vi "obj_DataLog Tag Meta Tags.vi"(0 "method":T3, 7 "point to write":T2 {"value" format="%.3e"; "time" format="%<%H:%M:%S%2u\n%Y/%m/%d>T"}, 9 "tag index in":i32=-1, 11 "error in (no error)":errorcluster) -> (4 "limit events":T1[](array[typedef]), 6 "exceeded mask":u32 format="%.0b", 8 "meta tag indices (-1 if none)":i32[](array[numeric]), 10 "tag index dup":i32, 15 "error out":errorcluster)   [LabVIEW 2012]
doc: "This object serves to apply meta tags to points being written to tags with direct valuation. Since only existing meta tags require application, the meta tags are collected on initialization so that their existence can be quickly determined. The max/min bounds are applied when exceeded. Subsequently, exceeded limits cause corresponding flags to be set, but the events are triggered conditionally based on the tag configuration settings intended to supress spurious events. Also, events are not handled by this non-reentrant object so as to prevent contention (event handling can be expensive). To ensure limit event handling, this object's {apply and write} method may not be called directly. Instead the \"Check and Write Point\" reentrant VI should be used since, in addition to calling {apply and write}, it implements event handling without contention.\n\nSince the {apply and write} method is called very frequently, some effort was put into minimizing its average overhead by putting most checking code on the same diagram (wich prevents subVI calling overhead) as well as by deferring object calls as long as possible by first checking for necessity. Hence the rather large diagram."
uses:
  typedefs/t_DataLog Tag Meta Tags Methods.ctl
  typedefs/et_DataLog Meta Tag Specifier.ctl
  typedefs/clusters/t_DataLog Point.ctl
  typedefs/t_DataLog Tag Hash Methods.ctl
  typedefs/t_DataLog Tag Info List Methods.ctl
  typedefs/t_DataLog Tag Buffers Methods.ctl
  subvis/private/glb_DataLog Runtime Parameterisation.vi
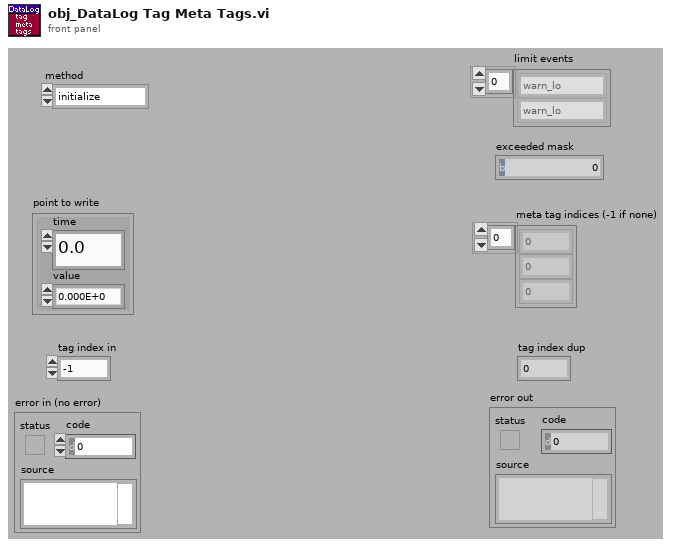
[diagram p1: front panel]
types:
  T1 = typedef "et_DataLog Meta Tag Specifier.ctl" = enum32{"warn_lo", "warn_hi", "A_lo", "A_hi", "B_lo", "B_hi", "C_lo", "C_hi", "D_lo", "D_hi", "E_lo", "E_hi", "F_lo", "F_hi", "G_lo", "G_hi", "H_lo", "H_hi", "I_lo", "I_hi", "J_lo", "J_hi", "K_lo", "K_hi", "L_lo", "L_hi", "M_lo", "M_hi", "N_lo", "N_hi", "min", "max", "not a meta"}
  T2 = typedef "t_DataLog Point.ctl" = cluster{"time":dbl, "value":dbl}
  T3 = typedef "t_DataLog Tag Meta Tags Methods.ctl" = enum16{"initialize", "apply and write", "get exceeded", "get metas", "cleanup"}
  T4 = typedef "t_DataLog Tag Hash Methods.ctl" = enum16{"initialize", "add tag", "index tag", "lookup", "#tags", "cleanup", "write recovery", "read recovery", "delete recovery"}
  T5 = typedef "t_DataLog Tag Info List Methods.ctl" = enum16{"initialize", "create", "create empty", "rename", "delete", "test tag", "get", "get by name", "get default", "get list", "get path", "get subsets", "set subsets", "set config", "set capacity", "#tags", "go live", "set unlocked", "set mirrored"}
  T6 = typedef "t_DataLog Tag Buffers Methods.ctl" = enum16{"initialize", "inert", "write", "read", "read oldest", "read last", "cleanup"}
  T7 = typedef "t_DataLog Tag Config.ctl" = cluster{"name":string, "unit":string, "temporal":T8, "value":T9, "index":i32, "capacity":i32, "is meta?":bool, "mincapacity":i32, "deadband":dbl, "limit delay":dbl, "format":T10, "precision":u8, "undefine":bool, "update":bool, "update period":u16, "expression":string, "description":string, "logging algorithm":T11, "logging parameters":dbl[]}
  T8 = typedef "t_DataLog Temporal Types.ctl" = enum16{"set&hold", "sample", "event"}
  T9 = typedef "t_DataLog Value Types.ctl" = enum16{"number", "string"}
  T10 = typedef "t_DataLog Numerical Format.ctl" = enum8{"fractional", "exponential", "engineering"}
  T11 = typedef "t_DataLog Logging Algorithms.ctl" = enum16{"nothing", "changes", "everything", "every Nth", "time threshold", "value threshold + prior", "t or v threshold", "t or v threshold + prior"}
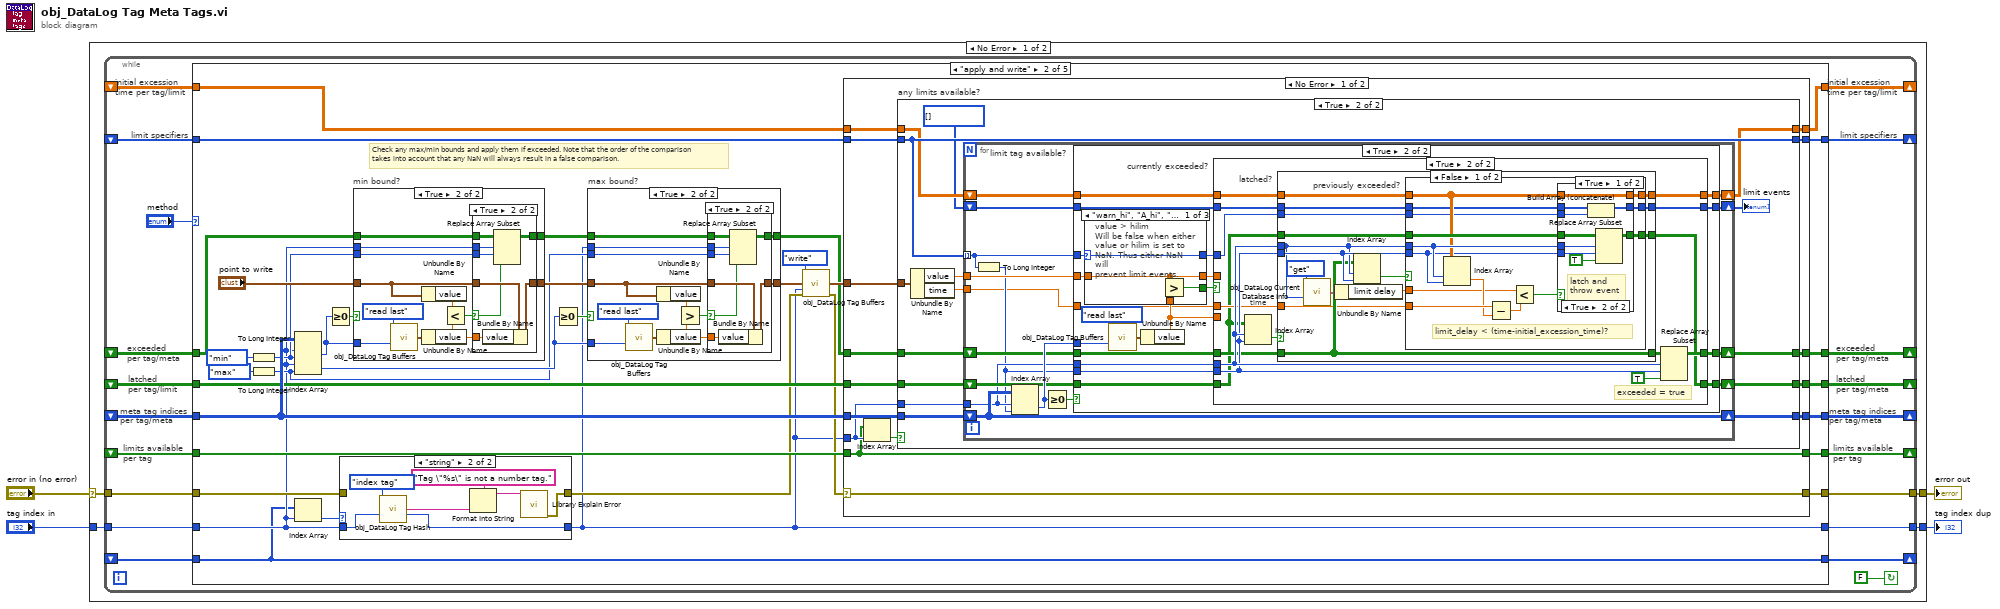
[diagram p0: block diagram]
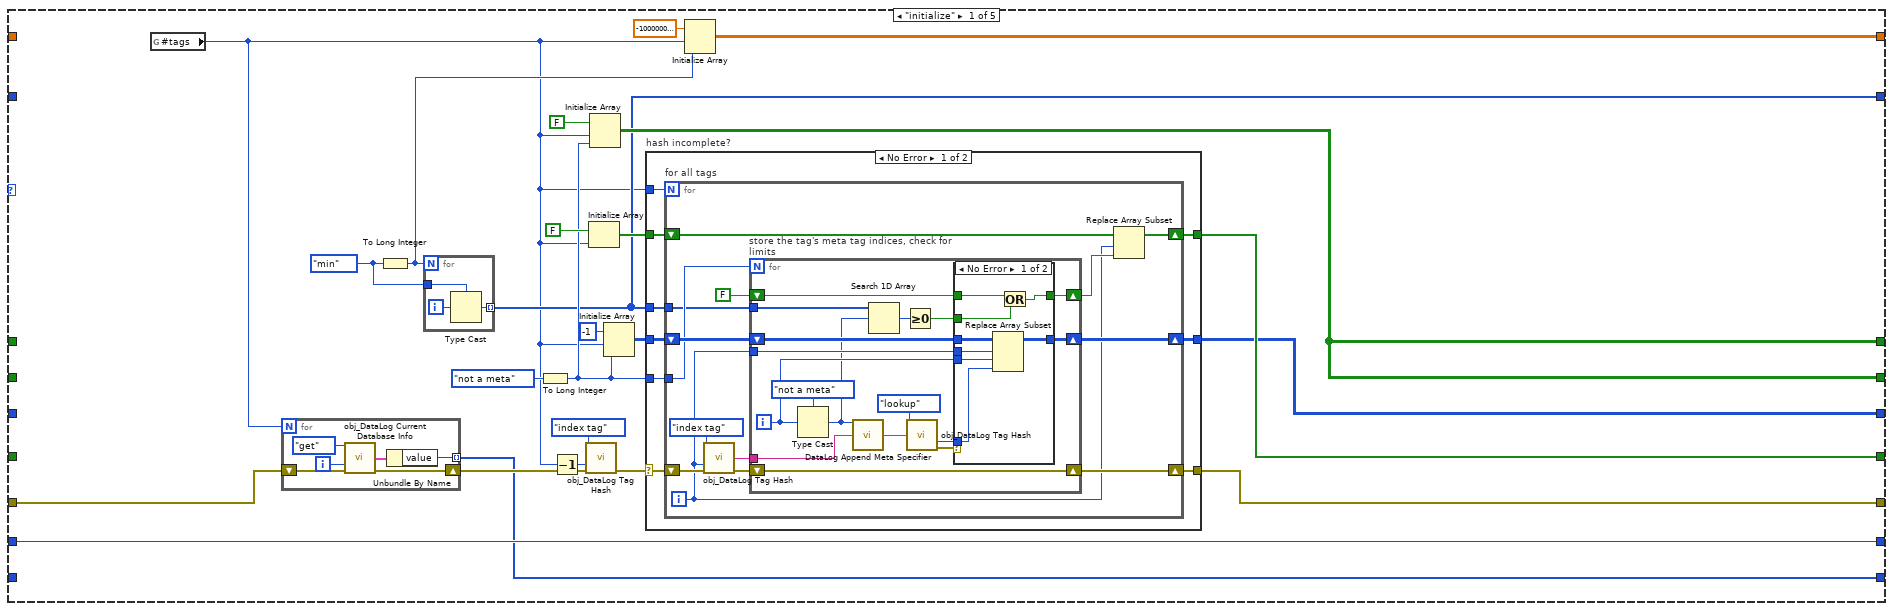
[diagram p2: hidden frame]
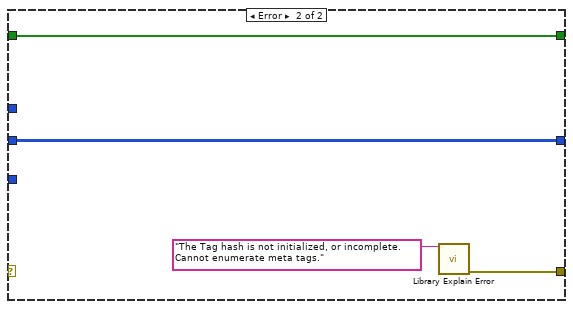
[diagram p4: hidden frame]
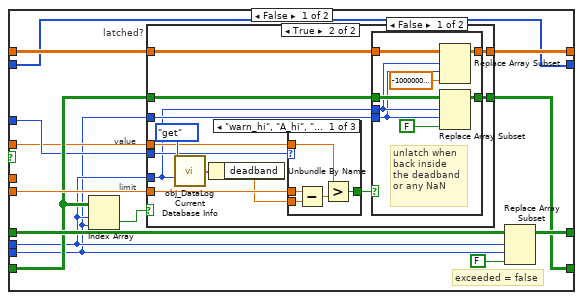
[diagram p8: hidden frame]
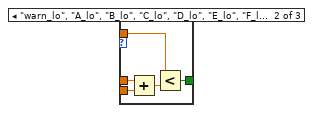
[diagram p11: hidden frame]
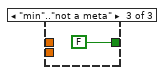
[diagram p12: hidden frame]
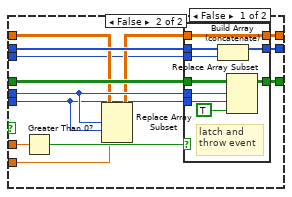
[diagram p14: hidden frame]
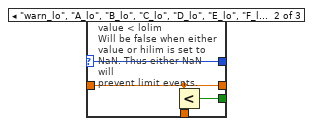
[diagram p17: hidden frame]
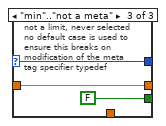
[diagram p18: hidden frame]
diagram:
  n1 = case shown="No Error" "error in (no error)" {
    selector: "error in (no error)" -> [w8 w581]
    tunnel: [w7 w581] -> w3
    tunnel: [w6 w580] -> w2
    tunnel: "tag index in" -> [w5 w580]
    frame No Error {
      n2 = while {
        shift-right: [w26] -> _
        shift-left: _ -> [w25]
        tunnel: w8 -> [w24]
        tunnel: [w23] -> w7
        shift-right: [w21] -> _
        shift-left: _ -> [w22]
        shift-right: [w19] -> _
        shift-left: _ -> [w20]
        shift-right: [w17] -> _
        shift-left: _ -> [w18]
        shift-right: [w15] -> _
        shift-left: _ -> [w16]
        shift-right: [w14] -> _
        shift-left: _ -> [w13]
        shift-right: [w12] -> _
        shift-left: _ -> [w11]
        tunnel: [w10] -> w6
        tunnel: w5 -> [w9]
        stop <- FALSE continue-if-true
        # "initial excession\ntime per tag/limit"
        # "limit specifiers"
        # "limits available\nper tag"
        # "exceeded\nper tag/meta"
        # "latched\nper tag/meta"
        # "meta tag indices\nper tag/meta"
        # "exceeded\nper tag/meta"
        # "latched\nper tag/meta"
        # "exceeded\nper tag/meta"
        # "initial excession\ntime per tag/limit"
        # "exceeded\nper tag/meta"
        # "limit specifiers"
        # "latched\nper tag/limit"
        # "limits available\nper tag"
        # "meta tag indices\nper tag/meta"
        n3 = case shown="\"apply and write\"" "method" {
          tunnel: w25 -> [_ w149 w456 w536 w571]
          tunnel: [w48 w148 w449 w529 w568] -> w26
          tunnel: w24 -> [w31 w121 w458 w538 w579]
          tunnel: [w51 w132 w460 w540 w579] -> w23
          tunnel: w22 -> [_ w150 w447 w527 w573]
          tunnel: [w50 w131 w457 w537 w572] -> w21
          tunnel: w20 -> [_ w146 w452 w532 w570]
          tunnel: [w39 w147 w455 w535 w569] -> w19
          tunnel: w9 -> [w41 w118 w454 w534 w578]
          tunnel: [w41 w119 w453 w533 w578] -> w10
          tunnel: w18 -> [_ w145 w446 w526 w577]
          tunnel: [w35 w144 w445 w526 w575] -> w17
          tunnel: w16 -> [_ w126 w451 w531 w564]
          tunnel: [w39 w130 w450 w530 w563] -> w15
          tunnel: [w38 w142 w448 w528 w561] -> w14
          tunnel: w13 -> [_ w143 w448 w528 w562]
          tunnel: [w29 w117 w444 w525 w557] -> w12
          tunnel: w11 -> [_ w117 w444 w525 w558]
          frame "initialize" {
            w34 = et_DataLog_Meta_Tag_Specifier."min" ("meta specifier")
            n4 = global read "glb_DataLog Runtime Parameterisation.vi" "#tags"() -> (w32:i32)
            n5 = for {
              N: w32 -> [_]
              shift-right: [w54] -> w30
              shift-left: w31 -> [w55]
              tunnel: [w53] -> w29 mode=indexing
              i -> [w56]
              n6 = call "obj_DataLog Current Database Info.vi"("method"=t_DataLog_Tag_Info_List_Methods."get", "tag index/change#"=w56, "error in (no error)"=w55) -> ("tag config out"=w57:T7, "error out"=w54:errorcluster)  [unwired: 6 in, 5 out]
              n7 = Unbundle By Name(w57) -> ("value"=w53:T9)
            }
            n8 = To Long Integer(number=w34) -> (32bit integer=w33:i32)
            n9 = for {
              N: w33 -> [_]
              tunnel: w34 -> [w61]
              tunnel: [w59] -> w35 mode=indexing
              i -> [w60]
              n10 = Type Cast(type=w61, x=w60) -> (*(type *) &x=w59:T1)
            }
            n11 = To Long Integer(number=et_DataLog_Meta_Tag_Specifier."not a meta" ("limit specifier")) -> (32bit integer=w36:i32)
            n12 = Decrement(x=w32) -> (x-1=w47:i32)
            n13 = call "obj_DataLog Tag Hash.vi"("method"=t_DataLog_Tag_Hash_Methods."index tag", "tag index in"=w47, "error in (no error)"=w30) -> ("error out"=w45:errorcluster)  [unwired: 9 in, 3 out]
            n14 = Initialize Array(FALSE, w32) -> (w49:bool[])
            n15 = Initialize Array(FALSE, w32, w36) -> (w39:bool[][])
            n16 = Initialize Array(-1 ("warning lolim"), w32, w36) -> (w43:i32[][])
            n17 = case "hash incomplete?" shown="No Error" w45 {
              selector: w45 -> [w64 _]
              tunnel: w32 -> [w70 _]
              tunnel: [w65 w112] -> w51
              tunnel: [w69 w115] -> w50
              tunnel: w49 -> [w68 w115]
              tunnel: [w67 w114] -> w48
              tunnel: w43 -> [w66 w114]
              tunnel: w36 -> [w63 _]
              tunnel: w35 -> [w62 _]
              frame No Error {
                n18 = for "for all tags" {
                  N: w70 -> [_]
                  shift-right: [w78] -> w69
                  shift-left: w68 -> [w77]
                  shift-right: [w75] -> w67
                  shift-left: w66 -> [w76]
                  shift-right: [w81] -> w65
                  shift-left: w64 -> [w83]
                  tunnel: w63 -> [w74]
                  tunnel: w62 -> [w71]
                  i -> [w72]
                  n19 = call "obj_DataLog Tag Hash.vi"("method"=t_DataLog_Tag_Hash_Methods."index tag", "tag index in"=w72, "error in (no error)"=w83) -> ("tag out"=w80:string, "error out"=w82:errorcluster)  [unwired: 9 in, 2 out]
                  n20 = for "store the tag's meta tag indices, check for limits" {
                    N: w74 -> [_]
                    shift-right: [w86] -> w81
                    shift-left: w82 -> [w86]
                    tunnel: w80 -> [w97]
                    shift-right: [w100] -> w75
                    shift-left: w76 -> [w101]
                    shift-right: [w98] -> w73
                    shift-left: FALSE -> [w99]
                    tunnel: w72 -> [w91]
                    tunnel: w71 -> [w89]
                    i -> [w90]
                    n21 = Type Cast(type=et_DataLog_Meta_Tag_Specifier."not a meta" ("limit specifier"), x=w90) -> (*(type *) &x=w85:T1)
                    n22 = call "DataLog Append Meta Specifier.vi"("meta specifier"=w85, "tag in"=w97) -> ("tag out"=w95:string)  [unwired: 13 in]
                    n23 = Search 1D Array(1D array=w89, element=w85) -> (index of element=w88:i32)  [unwired: 1 in]
                    n24 = Greater Or Equal To 0?(x=w88) -> (x >= 0?=w87:bool)
                    n25 = call "obj_DataLog Tag Hash.vi"("method"=t_DataLog_Tag_Hash_Methods."lookup", "tag in"=w95) -> ("tag index out"=w93:i32, "error out"=w92:errorcluster)  [unwired: 10 in, 2 out]
                    n26 = case shown="No Error" w92 {
                      tunnel: w101 -> [w108 w110]
                      tunnel: [w107 w110] -> w100
                      tunnel: w99 -> [w103 w111]
                      tunnel: [w109 w111] -> w98
                      tunnel: w93 -> [w106 _]
                      tunnel: w91 -> [w105 _]
                      tunnel: w90 -> [w104 _]
                      tunnel: w87 -> [w102 _]
                      frame No Error {
                        n27 = Replace Array Subset(array=w108, new element=w106, index (row)=w105, index (col)=w104) -> (w107:i32[][])
                        n28 = Or(x=w103, y=w102) -> (x .or. y?=w109:bool)
                      }
                      frame Error {
                      }
                    }
                  }
                  n29 = Replace Array Subset(array=w77, new element=w73, index=w72) -> (w78:bool[])
                }
              }
              frame Error {
                n30 = call "Library Explain Error.vi"("explanation prefix (none)"="The Tag hash is not initialized, or incomplete. Cannot enumerate meta tags." ("explanation")) -> ("explained error"=w112:errorcluster)  [unwired: 14 in]
              }
            }
            n31 = Initialize Array(-1000000000000.0, w32, w33) -> (w38:dbl[][])
          }
          frame "apply and write" {
            # "Check any max/min bounds and apply them if exceeded. Note that the order of the comparison takes into account that any NaN will always result in a false comparison."
            n32 = To Long Integer(number=et_DataLog_Meta_Tag_Specifier."min" ("meta specifier")) -> (32bit integer=w122:i32)
            n33 = To Long Integer(number=et_DataLog_Meta_Tag_Specifier."max" ("meta specifier")) -> (32bit integer=w125:i32)
            n34 = Index Array(array=w149, index (row) #1=w118, index (col) #1=w122, index (row) #2=w118, index (col) #2=w125) -> (element #1=w137:i32, element #2=w129:i32)
            n35 = Index Array(array=w117, index=w118) -> (element=w116:T9)
            n36 = Greater Or Equal To 0?(x=w137) -> (x >= 0?=w136:bool)
            n37 = case shown="\"string\"" w116 {
              tunnel: w121 -> [w152 _]
              tunnel: [w152 w155] -> w120
              tunnel: w118 -> [w151 w154]
              tunnel: [w151 w153] -> w119
              frame "number" {
              }
              frame "string" {
                n38 = call "obj_DataLog Tag Hash.vi"("method"=t_DataLog_Tag_Hash_Methods."index tag", "tag index in"=w154) -> ("tag out"=w156:string, "tag index out"=w153:i32)  [unwired: 10 in, 2 out]
                n39 = Format Into String(format string="Tag \"%s\" is not a number tag.", w156) -> (resulting string=w157:string)  [unwired: 2 in, 1 out]
                n40 = call "Library Explain Error.vi"("explanation prefix (none)"=w157) -> ("explained error"=w155:errorcluster)  [unwired: 14 in]
              }
            }
            n41 = case "min bound?" shown="True" w136 {
              tunnel: w137 -> [_ w427]
              tunnel: "point to write" -> [w417 w423]
              tunnel: [w417 w422] -> w128
              tunnel: w126 -> [w416 w421]
              tunnel: w118 -> [_ w420]
              tunnel: [w416 w419] -> w124
              tunnel: w122 -> [_ w418]
              frame False {
              }
              frame True {
                n42 = call "obj_DataLog Tag Buffers.vi"("method"=t_DataLog_Tag_Buffers_Methods."read last", "tag index"=w427) -> ("point out"=w429:T2)  [unwired: 9 in, 4 out]
                n43 = Unbundle By Name(w423) -> ("value"=w426:dbl)
                n44 = Unbundle By Name(w429) -> ("value"=w425:dbl)
                n45 = Less?(x=w426, y=w425) -> (x < y?=w424:bool)
                n46 = case shown="True" w424 {
                  selector: w424 -> [w433 w436]
                  tunnel: w423 -> [w435 w443]
                  tunnel: w425 -> [_ w441]
                  tunnel: [w435 w442] -> w422
                  tunnel: w421 -> [w434 w440]
                  tunnel: w420 -> [w431 w439]
                  tunnel: [w430 w438] -> w419
                  tunnel: w418 -> [w432 w437]
                  frame False {
                    n47 = Replace Array Subset(array=w434, new element=w433, index (row)=w431, index (col)=w432) -> (w430:bool[][])
                  }
                  frame True {
                    n48 = Bundle By Name(cluster=w443, "value"=w441) -> (w442:T2)
                    n49 = Replace Array Subset(array=w440, new element=w436, index (row)=w439, index (col)=w437) -> (w438:bool[][])
                  }
                }
              }
            }
            n50 = Greater Or Equal To 0?(x=w129) -> (x >= 0?=w135:bool)
            n51 = case "max bound?" shown="True" w135 {
              tunnel: w129 -> [_ w399]
              tunnel: w128 -> [w389 w395]
              tunnel: [w389 w394] -> w134
              tunnel: w119 -> [_ w393]
              tunnel: w124 -> [w388 w392]
              tunnel: w125 -> [_ w391]
              tunnel: [w388 w390] -> w123
              frame False {
              }
              frame True {
                n52 = call "obj_DataLog Tag Buffers.vi"("method"=t_DataLog_Tag_Buffers_Methods."read last", "tag index"=w399) -> ("point out"=w401:T2)  [unwired: 9 in, 4 out]
                n53 = Unbundle By Name(w395) -> ("value"=w398:dbl)
                n54 = Unbundle By Name(w401) -> ("value"=w397:dbl)
                n55 = Greater?(x=w398, y=w397) -> (0:w396:bool)
                n56 = case shown="True" w396 {
                  selector: w396 -> [w403 w411]
                  tunnel: w395 -> [w407 w415]
                  tunnel: w397 -> [_ w413]
                  tunnel: [w407 w414] -> w394
                  tunnel: w393 -> [w405 w412]
                  tunnel: w392 -> [w406 w410]
                  tunnel: w391 -> [w404 w409]
                  tunnel: [w402 w408] -> w390
                  frame False {
                    n57 = Replace Array Subset(array=w406, new element=w403, index (row)=w405, index (col)=w404) -> (w402:bool[][])
                  }
                  frame True {
                    n58 = Bundle By Name(cluster=w415, "value"=w413) -> (w414:T2)
                    n59 = Replace Array Subset(array=w410, new element=w411, index (row)=w412, index (col)=w409) -> (w408:bool[][])
                  }
                }
              }
            }
            n60 = call "obj_DataLog Tag Buffers.vi"("method"=t_DataLog_Tag_Buffers_Methods."write", "point in"=w134, "tag index"=w119, "error in (no error)"=w120) -> ("point out"=w140:T2, "error out"=w133:errorcluster)  [unwired: 7 in, 3 out]
            n61 = case shown="No Error" w133 {
              selector: w133 -> [w162 w387]
              tunnel: w150 -> [w161 w386]
              tunnel: w149 -> [w174 w385]
              tunnel: [w173 w385] -> w148
              tunnel: [w172 w384] -> w147
              tunnel: w146 -> [w171 w384]
              tunnel: w123 -> [w170 w381]
              tunnel: w145 -> [w169 w382]
              tunnel: [w168 w382] -> w144
              tunnel: w143 -> [w167 w383]
              tunnel: [w166 w383] -> w142
              tunnel: w119 -> [w165 _]
              tunnel: w140 -> [w163 _]
              tunnel: [w162 w387] -> w132
              tunnel: [w161 w386] -> w131
              tunnel: [w160 w381] -> w130
              frame No Error {
                n62 = Index Array(array=w161, index=w165) -> (element=w164:bool)
                n63 = case "any limits available?" shown="True" w164 {
                  tunnel: w174 -> [w178 w193]
                  tunnel: w171 -> [w179 w188]
                  tunnel: w163 -> [_ w194]
                  tunnel: [w179 w186] -> w172
                  tunnel: [w178 w192] -> w173
                  tunnel: w165 -> [_ w189]
                  tunnel: w169 -> [w177 w190]
                  tunnel: [w177 w190] -> w168
                  tunnel: w170 -> [w175 w187]
                  tunnel: w167 -> [w176 w183]
                  tunnel: [w176 w182] -> w166
                  tunnel: [w175 w185] -> w160
                  frame False {
                  }
                  frame True {
                    w181 = T1[] [] items=["warn_lo", "warn_hi", "A_lo", "A_hi", "B_lo", "B_hi", "C_lo", "C_hi", "D_lo", "D_hi", "E_lo", "E_hi", "F_lo", "F_hi", "G_lo", "G_hi", "H_lo", "H_hi", "I_lo", "I_hi", "J_lo", "J_hi", "K_lo", "K_hi", "L_lo", "L_hi", "M_lo", "M_hi", "N_lo", "N_hi", "min", "max", "not a meta"] ("limit events")
                    n64 = Unbundle By Name(w194) -> ("value"=w184:dbl, "time"=w191:dbl)
                    n65 = for {
                      shift-right: [w210] -> w192
                      shift-left: w193 -> [w210]
                      tunnel: w191 -> [w197]
                      tunnel: w190 -> [w207] mode=indexing
                      tunnel: w189 -> [w199]
                      shift-right: [w200] -> w186
                      shift-left: w188 -> [w206]
                      shift-right: [w201] -> w185
                      shift-left: w187 -> [w204]
                      tunnel: w184 -> [w205]
                      shift-right: [w202] -> w182
                      shift-left: w183 -> [w203]
                      shift-right: [w195] -> w180
                      shift-left: w181 -> [w196]
                      n66 = To Long Integer(number=w207) -> (32bit integer=w198:i32)
                      n67 = Index Array(array=w210, index (row)=w199, index (col)=w198) -> (element=w209:i32)
                      n68 = Greater Or Equal To 0?(x=w209) -> (x >= 0?=w208:bool)
                      n69 = case "limit tag available?" shown="True" w208 {
                        tunnel: w207 -> [_ w231]
                        tunnel: w209 -> [_ w234]
                        tunnel: w206 -> [w212 w227]
                        tunnel: w205 -> [_ w230]
                        tunnel: w204 -> [w213 w228]
                        tunnel: w203 -> [w214 w226]
                        tunnel: [w214 w225] -> w202
                        tunnel: [w213 w224] -> w201
                        tunnel: [w212 w221] -> w200
                        tunnel: w199 -> [_ w223]
                        tunnel: w198 -> [_ w222]
                        tunnel: w197 -> [_ w217]
                        tunnel: w196 -> [w211 w216]
                        tunnel: [w211 w215] -> w195
                        frame False {
                        }
                        frame True {
                          n70 = call "obj_DataLog Tag Buffers.vi"("method"=t_DataLog_Tag_Buffers_Methods."read last", "tag index"=w234) -> ("point out"=w232:T2)  [unwired: 9 in, 4 out]
                          n71 = Unbundle By Name(w232) -> ("value"=w219:dbl)
                          n72 = case shown="\"warn_hi\", \"A_hi\", \"B_hi\", \"C_hi\", \"D_hi\", \"E_hi\", \"F_hi\", \"G_hi\", \"H_hi\", \"I_hi\", \"J_hi\", \"K_hi\", \"L_hi\", \"M_hi\", \"N_hi\"" w231 {
                            selector: w231 -> [w370 w374 w378]
                            tunnel: w230 -> [w371 w375 w379]
                            tunnel: w219 -> [w373 w377 _]
                            tunnel: [w372 w376 FALSE] -> w229
                            tunnel: [w371 w375 w379] -> w220
                            tunnel: [w370 w374 w378] -> w218
                            frame "warn_hi", "A_hi", "B_hi", "C_hi", "D_hi", "E_hi", "F_hi", "G_hi", "H_hi", "I_hi", "J_hi", "K_hi", "L_hi", "M_hi", "N_hi" {
                              # "value > hilim\nWill be false when either value or hilim is set to NaN. Thus either NaN will\nprevent limit events."
                              n73 = Greater?(x=w371, y=w373) -> (0:w372:bool)
                            }
                            frame "warn_lo", "A_lo", "B_lo", "C_lo", "D_lo", "E_lo", "F_lo", "G_lo", "H_lo", "I_lo", "J_lo", "K_lo", "L_lo", "M_lo", "N_lo" {
                              # "value < lolim\nWill be false when either value or hilim is set to NaN. Thus either NaN will\nprevent limit events."
                              n74 = Less?(x=w375, y=w377) -> (x < y?=w376:bool)
                            }
                            frame "min".."not a meta" {
                              # "not a limit, never selected\nno default case is used to\nensure this breaks on modification of the meta\ntag specifier typedef"
                            }
                          }
                          n75 = case "currently exceeded?" shown="True" w229 {
                            tunnel: w228 -> [w248 w287]
                            tunnel: w227 -> [w243 w285]
                            tunnel: w226 -> [w236 w293]
                            tunnel: [w237 w292] -> w225
                            tunnel: [w247 w299] -> w224
                            tunnel: w223 -> [w241 w295]
                            tunnel: w222 -> [w238 w294]
                            tunnel: [w242 w296] -> w221
                            tunnel: w220 -> [w239 _]
                            tunnel: w219 -> [w244 _]
                            tunnel: w218 -> [w240 w289]
                            tunnel: w217 -> [_ w291]
                            tunnel: w216 -> [w235 w290]
                            tunnel: [w235 w288] -> w215
                            frame False {
                              # "exceeded = false"
                              # "limit"
                              # "value"
                              n76 = Index Array(array=w243, index (row)=w241, index (col)=w238) -> (element=w245:bool)
                              n77 = case "latched?" shown="True" w245 {
                                tunnel: w244 -> [_ w259]
                                tunnel: w243 -> [w250 w256]
                                tunnel: [w250 w255] -> w242
                                tunnel: w241 -> [_ w253]
                                tunnel: w240 -> [_ w261]
                                tunnel: w239 -> [_ w260]
                                tunnel: w238 -> [_ w254]
                                tunnel: [w249 w252] -> w237
                                tunnel: w236 -> [w249 w251]
                                frame False {
                                }
                                frame True {
                                n78 = call "obj_DataLog Current Database Info.vi"("method"=t_DataLog_Tag_Info_List_Methods."get", "tag index/change#"=w253) -> ("tag config out"=w262:T7)  [unwired: 7 in, 6 out]
                                n79 = Unbundle By Name(w262) -> ("deadband"=w258:dbl)
                                n80 = case shown="\"warn_hi\", \"A_hi\", \"B_hi\", \"C_hi\", \"D_hi\", \"E_hi\", \"F_hi\", \"G_hi\", \"H_hi\", \"I_hi\", \"J_hi\", \"K_hi\", \"L_hi\", \"M_hi\", \"N_hi\"" w261 {
                                tunnel: [w278 w283 FALSE] -> w257
                                tunnel: w260 -> [w274 w282 _]
                                tunnel: w259 -> [w276 w280 _]
                                tunnel: w258 -> [w277 w279 _]
                                frame "warn_hi", "A_hi", "B_hi", "C_hi", "D_hi", "E_hi", "F_hi", "G_hi", "H_hi", "I_hi", "J_hi", "K_hi", "L_hi", "M_hi", "N_hi" {
                                n81 = Subtract(x=w276, y=w277) -> (x-y=w275:dbl)
                                n82 = Greater?(x=w274, y=w275) -> (0:w278:bool)
                                }
                                frame "warn_lo", "A_lo", "B_lo", "C_lo", "D_lo", "E_lo", "F_lo", "G_lo", "H_lo", "I_lo", "J_lo", "K_lo", "L_lo", "M_lo", "N_lo" {
                                n83 = Add(x=w280, y=w279) -> (x+y=w281:dbl)
                                n84 = Less?(x=w282, y=w281) -> (x < y?=w283:bool)
                                }
                                frame "min".."not a meta" {
                                }
                                }
                                n85 = case shown="False" w257 {
                                tunnel: w256 -> [w270 w273]
                                tunnel: [w269 w273] -> w255
                                tunnel: w254 -> [w265 _]
                                tunnel: w253 -> [w266 _]
                                tunnel: [w268 w272] -> w252
                                tunnel: w251 -> [w267 w272]
                                frame False {
                                # "unlatch when\nback inside\nthe deadband\nor any NaN"
                                n86 = Replace Array Subset(array=w267, new element=-1000000000000.0, index (row)=w266, index (col)=w265) -> (w268:dbl[][])
                                n87 = Replace Array Subset(array=w270, new element=FALSE ("new element/subarray"), index (row)=w266, index (col)=w265) -> (w269:bool[][])
                                }
                                frame True {
                                }
                                }
                                }
                              }
                              n88 = Replace Array Subset(array=w248, new element=FALSE ("new element/subarray"), index (row)=w241, index (col)=w238) -> (w247:bool[][])
                            }
                            frame True {
                              # "exceeded = true"
                              # "time"
                              n89 = Index Array(array=w285, index (row)=w295, index (col)=w294) -> (element=w297:bool)
                              n90 = case "latched?" shown="False" w297 {
                                tunnel: w285 -> [w309 w369]
                                tunnel: [w313 w369] -> w296
                                tunnel: w295 -> [w311 _]
                                tunnel: w294 -> [w312 _]
                                tunnel: w293 -> [w306 w368]
                                tunnel: [w303 w368] -> w292
                                tunnel: w291 -> [w305 _]
                                tunnel: w290 -> [w302 w367]
                                tunnel: w289 -> [w300 _]
                                tunnel: [w301 w367] -> w288
                                tunnel: w287 -> [w308 w366]
                                tunnel: [w308 w366] -> w286
                                frame False {
                                n91 = call "obj_DataLog Current Database Info.vi"("method"=t_DataLog_Tag_Info_List_Methods."get", "tag index/change#"=w311) -> ("tag config out"=w307:T7)  [unwired: 7 in, 6 out]
                                n92 = Unbundle By Name(w307) -> ("limit delay"=w304:dbl)
                                n93 = Index Array(array=w308, index (row)=w311, index (col)=w312) -> (element=w310:bool)
                                n94 = case "previously exceeded?" shown="True" w310 {
                                tunnel: [w328 w353] -> w313
                                tunnel: w312 -> [w315 w341]
                                tunnel: w311 -> [w326 w346]
                                tunnel: w309 -> [w327 w352]
                                tunnel: w306 -> [w319 w344]
                                tunnel: w305 -> [w325 w345]
                                tunnel: w304 -> [w323 w348]
                                tunnel: [w320 w351] -> w303
                                tunnel: w302 -> [w318 w350]
                                tunnel: [w317 w349] -> w301
                                tunnel: w300 -> [w316 w342]
                                frame True {
                                # "limit_delay < (time-initial_excession_time)?"
                                n95 = Index Array(array=w319, index (row)=w326, index (col)=w315) -> (element=w324:dbl)
                                n96 = Subtract(x=w325, y=w324) -> (x-y=w322:dbl)
                                n97 = Less?(x=w323, y=w322) -> (x < y?=w321:bool)
                                n98 = case shown="True" w321 {
                                tunnel: w327 -> [w331 w339]
                                tunnel: [w331 w338] -> w328
                                tunnel: w315 -> [_ w337]
                                tunnel: w326 -> [_ w336]
                                tunnel: [w330 w335] -> w320
                                tunnel: w319 -> [w330 w335]
                                tunnel: w318 -> [w329 w334]
                                tunnel: [w329 w333] -> w317
                                tunnel: w316 -> [_ w332]
                                frame False {
                                }
                                frame True {
                                # "latch and\nthrow event"
                                n99 = Build Array (concatenate)(w334, w332) -> (w333:T1[])
                                n100 = Replace Array Subset(array=w339, new element=TRUE ("new element/subarray"), index (row)=w336, index (col)=w337) -> (w338:bool[][])
                                }
                                }
                                }
                                frame False {
                                n101 = Greater Than 0?(x=w348) -> (x > 0?=w347:bool)
                                n102 = Replace Array Subset(array=w344, new element=w345, index (row)=w346, index (col)=w341) -> (w343:dbl[][])
                                n103 = case shown="False" w347 {
                                tunnel: w352 -> [w361 w365]
                                tunnel: [w360 w365] -> w353
                                tunnel: w341 -> [w359 _]
                                tunnel: w346 -> [w358 _]
                                tunnel: [w357 w364] -> w351
                                tunnel: w343 -> [w357 w364]
                                tunnel: w350 -> [w356 w363]
                                tunnel: [w355 w363] -> w349
                                tunnel: w342 -> [w354 _]
                                frame False {
                                # "latch and\nthrow event"
                                n104 = Build Array (concatenate)(w356, w354) -> (w355:T1[])
                                n105 = Replace Array Subset(array=w361, new element=TRUE ("new element/subarray"), index (row)=w358, index (col)=w359) -> (w360:bool[][])
                                }
                                frame True {
                                }
                                }
                                }
                                }
                                }
                                frame True {
                                # "Limit already latched.\nNo need to throw\nanother event."
                                }
                              }
                              n106 = Replace Array Subset(array=w286, new element=TRUE ("new element/subarray"), index (row)=w295, index (col)=w294) -> (w299:bool[][])
                            }
                          }
                        }
                      }
                    }
                    "limit events" <- w180
                  }
                }
              }
              frame Error {
              }
            }
          }
          frame "get exceeded" {
            n107 = Array Size(array=w447) -> (size(s)=w462:i32)
            n108 = In Range and Coerce(upper limit=w462, x=w454, lower limit=0) -> (In Range?=w459:bool)  [unwired: 1 out]
            n109 = case "index in range?" shown="True" w459 {
              tunnel: w456 -> [w476 w519]
              tunnel: [w480 w524] -> w460
              tunnel: w458 -> [w480 _]
              tunnel: w447 -> [w482 w522]
              tunnel: [w482 w522] -> w457
              tunnel: w452 -> [w479 w520]
              tunnel: [w479 w520] -> w455
              tunnel: [w463 w521] -> w453
              tunnel: w454 -> [w463 w521]
              tunnel: w451 -> [w478 w518]
              tunnel: [w465 w518] -> w450
              tunnel: [w476 w519] -> w449
              tunnel: w446 -> [w475 w517]
              tunnel: [w474 w517] -> w445
              frame True {
                n110 = Index Array(array=w482, index=w463) -> (element=w481:bool)
                n111 = case "limits available?" shown="True" w481 {
                  tunnel: w463 -> [_ w503]
                  tunnel: w478 -> [w497 w504]
                  tunnel: [w497 w502] -> w465
                  tunnel: [w496 w501] -> w472
                  tunnel: u32 0 ("exceeded bits") -> [w496 w500]
                  tunnel: w475 -> [w495 w498]
                  tunnel: [w495 w498] -> w474
                  frame False {
                  }
                  frame True {
                    n112 = Array Size(array=w498) -> (size(s)=w499:i32)
                    n113 = for {
                      N: w499 -> [_]
                      shift-right: [w506] -> w502
                      shift-left: w504 -> [w506]
                      shift-right: [w507] -> w501
                      shift-left: w500 -> [w508]
                      tunnel: w503 -> [w510]
                      i -> [w505]
                      n114 = Index Array(array=w506, index (row)=w510, index (col)=w505) -> (element=w509:bool)
                      n115 = case shown="True" w509 {
                        tunnel: w505 -> [_ w515]
                        tunnel: w508 -> [w511 w514]
                        tunnel: [w511 w512] -> w507
                        frame False {
                        }
                        frame True {
                          n116 = Logical Shift(y=w515, x=u32 1) -> (x << y=w513:u32)
                          n117 = Or(x=w514, y=w513) -> (x .or. y?=w512:u32)
                        }
                      }
                    }
                  }
                }
                n118 = To Long Integer(number=et_DataLog_Meta_Tag_Specifier."min" ("meta specifier")) -> (32bit integer=w471:i32)
                n119 = Index Array(array=w465, index (row)=w463, index (col)=w471) -> (element=w473:bool)
                n120 = case shown="True" w473 {
                  tunnel: w471 -> [_ w493]
                  tunnel: w472 -> [w489 w492]
                  tunnel: [w489 w490] -> w466
                  frame False {
                  }
                  frame True {
                    n121 = Logical Shift(y=w493, x=u32 1) -> (x << y=w491:u32)
                    n122 = Or(x=w492, y=w491) -> (x .or. y?=w490:u32)
                  }
                }
                n123 = To Long Integer(number=et_DataLog_Meta_Tag_Specifier."max" ("meta specifier")) -> (32bit integer=w468:i32)
                n124 = Index Array(array=w465, index (row)=w463, index (col)=w468) -> (element=w467:bool)
                n125 = case shown="True" w467 {
                  tunnel: w468 -> [_ w487]
                  tunnel: w466 -> [w483 w486]
                  tunnel: [w483 w484] -> w464
                  frame False {
                  }
                  frame True {
                    n126 = Logical Shift(y=w487, x=u32 1) -> (x << y=w485:u32)
                    n127 = Or(x=w486, y=w485) -> (x .or. y?=w484:u32)
                  }
                }
                "exceeded mask" <- w464
              }
              frame False {
                n128 = call "Library Explain Error.vi"("explanation prefix (none)"="Wrong or unwired tag index, or unitialized object." ("explanation")) -> ("explained error"=w524:errorcluster)  [unwired: 14 in]
              }
            }
          }
          frame "get metas" {
            n129 = Array Size(array=w527) -> (size(s)=w542:i32)
            n130 = In Range and Coerce(upper limit=w542, x=w534, lower limit=0) -> (In Range?=w539:bool)  [unwired: 1 out]
            n131 = case "index in range?" shown="True" w539 {
              tunnel: w536 -> [w547 w551]
              tunnel: [w549 w556] -> w540
              tunnel: w538 -> [w549 _]
              tunnel: w527 -> [w545 w554]
              tunnel: [w545 w554] -> w537
              tunnel: w532 -> [w548 w552]
              tunnel: [w548 w552] -> w535
              tunnel: [w546 w553] -> w533
              tunnel: w534 -> [w546 w553]
              tunnel: w531 -> [w544 w550]
              tunnel: [w544 w550] -> w530
              tunnel: [w547 w551] -> w529
              frame True {
                n132 = Index Array(array=w547, index (row)=w546) -> (element=→"meta tag indices (-1 if none)":i32[])  [unwired: 1 in]
              }
              frame False {
                n133 = call "Library Explain Error.vi"("explanation prefix (none)"="Wrong or unwired tag index, or unitialized object." ("explanation")) -> ("explained error"=w556:errorcluster)  [unwired: 14 in]
              }
            }
          }
          frame "cleanup" {
            w560 = 0 ("dimension size")
            w565 = 0 ("dimension size")
            w566 = 0 ("dimension size")
            w567 = 0 ("dimension size")
            n134 = Reshape Array(w562, w560, w560) -> (w561:dbl[][])
            n135 = Reshape Array(w577, 0 ("dimension size")) -> (w575:T1[])
            n136 = Reshape Array(w564, w565, w565) -> (w563:bool[][])
            n137 = Reshape Array(w570, w566, w566) -> (w569:bool[][])
            n138 = Reshape Array(w571, w567, w567) -> (w568:i32[][])
            n139 = Reshape Array(w573, 0 ("dimension size")) -> (w572:bool[])
            n140 = Reshape Array(w558, 0 ("dimension size")) -> (w557:T9[])
          }
        }
      }
    }
    frame Error {
    }
  }
  "error out" <- w3
  "tag index dup" <- w2
